vi "Save CRT data to file.vi"(5 "GPS data granularity (minutes)":refnum<vi>, 6 "Hitrate save info":T2, 7 "ROB data granularity (minutes)":refnum<vi>, 8 "error in":errorcluster, 9 "Run ID":refnum<vi>, 10 "ROB Info cluster":refnum<vi>, 11 "HDF5 data file":refnum<vi>) -> (0 "error out":errorcluster)   [LabVIEW 2016]
uses:
  Typedefs/Hit chart cluster refnum.ctl
  Typedefs/CoincidencesToSave.ctl
  Typedefs/CoincidenceWithGPSformat.ctl
  Global Variables/take CRT data.vi
  <vilib>/addons/h5labview2/group/H5G.lvlib
  <vilib>/addons/h5labview2/dataset/H5D.lvlib
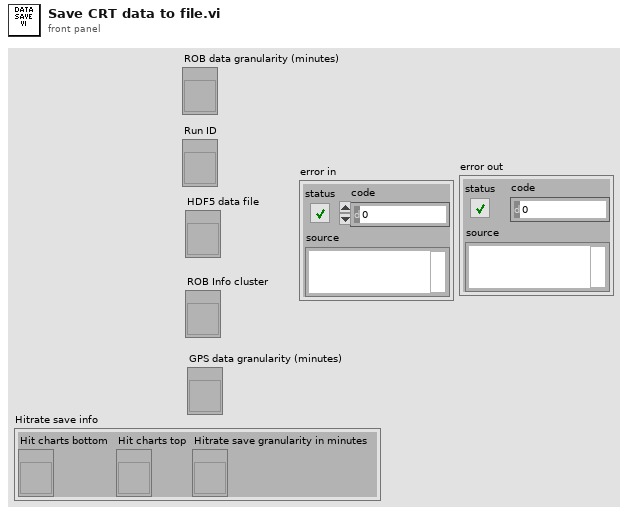
[diagram p1: front panel]
types:
  T1 = typedef "Hit chart cluster refnum.ctl" = refnum<vi>
  T2 = cluster{"Hit charts bottom":T1, "Hit charts top":T1, "Hitrate save granularity in minutes":refnum<vi>}
  T3 = typedef "CoincidenceWithGPSformat.ctl" = cluster{"Low-res hit time":u32, "Hi-res hit time":u32, "Secondary ID":i8, "DeltaT":i32, "Primary ID":i8}
  T4 = typedef "CoincidencesToSave.ctl" = T3[]
  T5 = cluster{"Timestamp":u32, "Fix quality":i8, "Satelites":i8}
  T6 = enum16{"insertPPS", "insertUTC", "read", "initiate"}
  T7 = typedef "hid_t.ctl" = i32
  T8 = cluster{"Pixel":i8, "Hi res hit time":u32, "Low res hit time":u32, "DeltaT":i16}[]
  T9 = typedef "HitChart.ctl" = cluster{"Waveform Chart":cluster{"Coincidences":dbl, "Non-coincidences":dbl, "Ratio":dbl, "Total hits":dbl}[], "Last update timestamp":timestamp, "Resolution(s)":dbl, "nondisplayed coincs":i32, "nondisplayed noncoincs":i32, "Last upd":i64, "ID":i8}
  T10 = cluster{"Waveform Chart":T9, "Waveform Chart 2":T9, "Waveform Chart 3":T9, "Waveform Chart 4":T9, "Waveform Chart 5":T9, "Waveform Chart 6":T9, "Waveform Chart 7":T9, "Waveform Chart 8":T9}
  T11 = cluster{"timestamp":u32, "ch0":dbl, "ch1":dbl, "ch2":dbl, "ch3":dbl, "ch4":dbl, "ch5":dbl, "ch6":dbl, "ch7":dbl, "ch8":dbl, "ch9":dbl, "ch10":dbl, "ch11":dbl, "ch12":dbl, "ch13":dbl, "ch14":dbl, "ch15":dbl}[]
  T12 = cluster{"Timestamp":u32, "Fix quality":i8, "Satelites":i8}[]
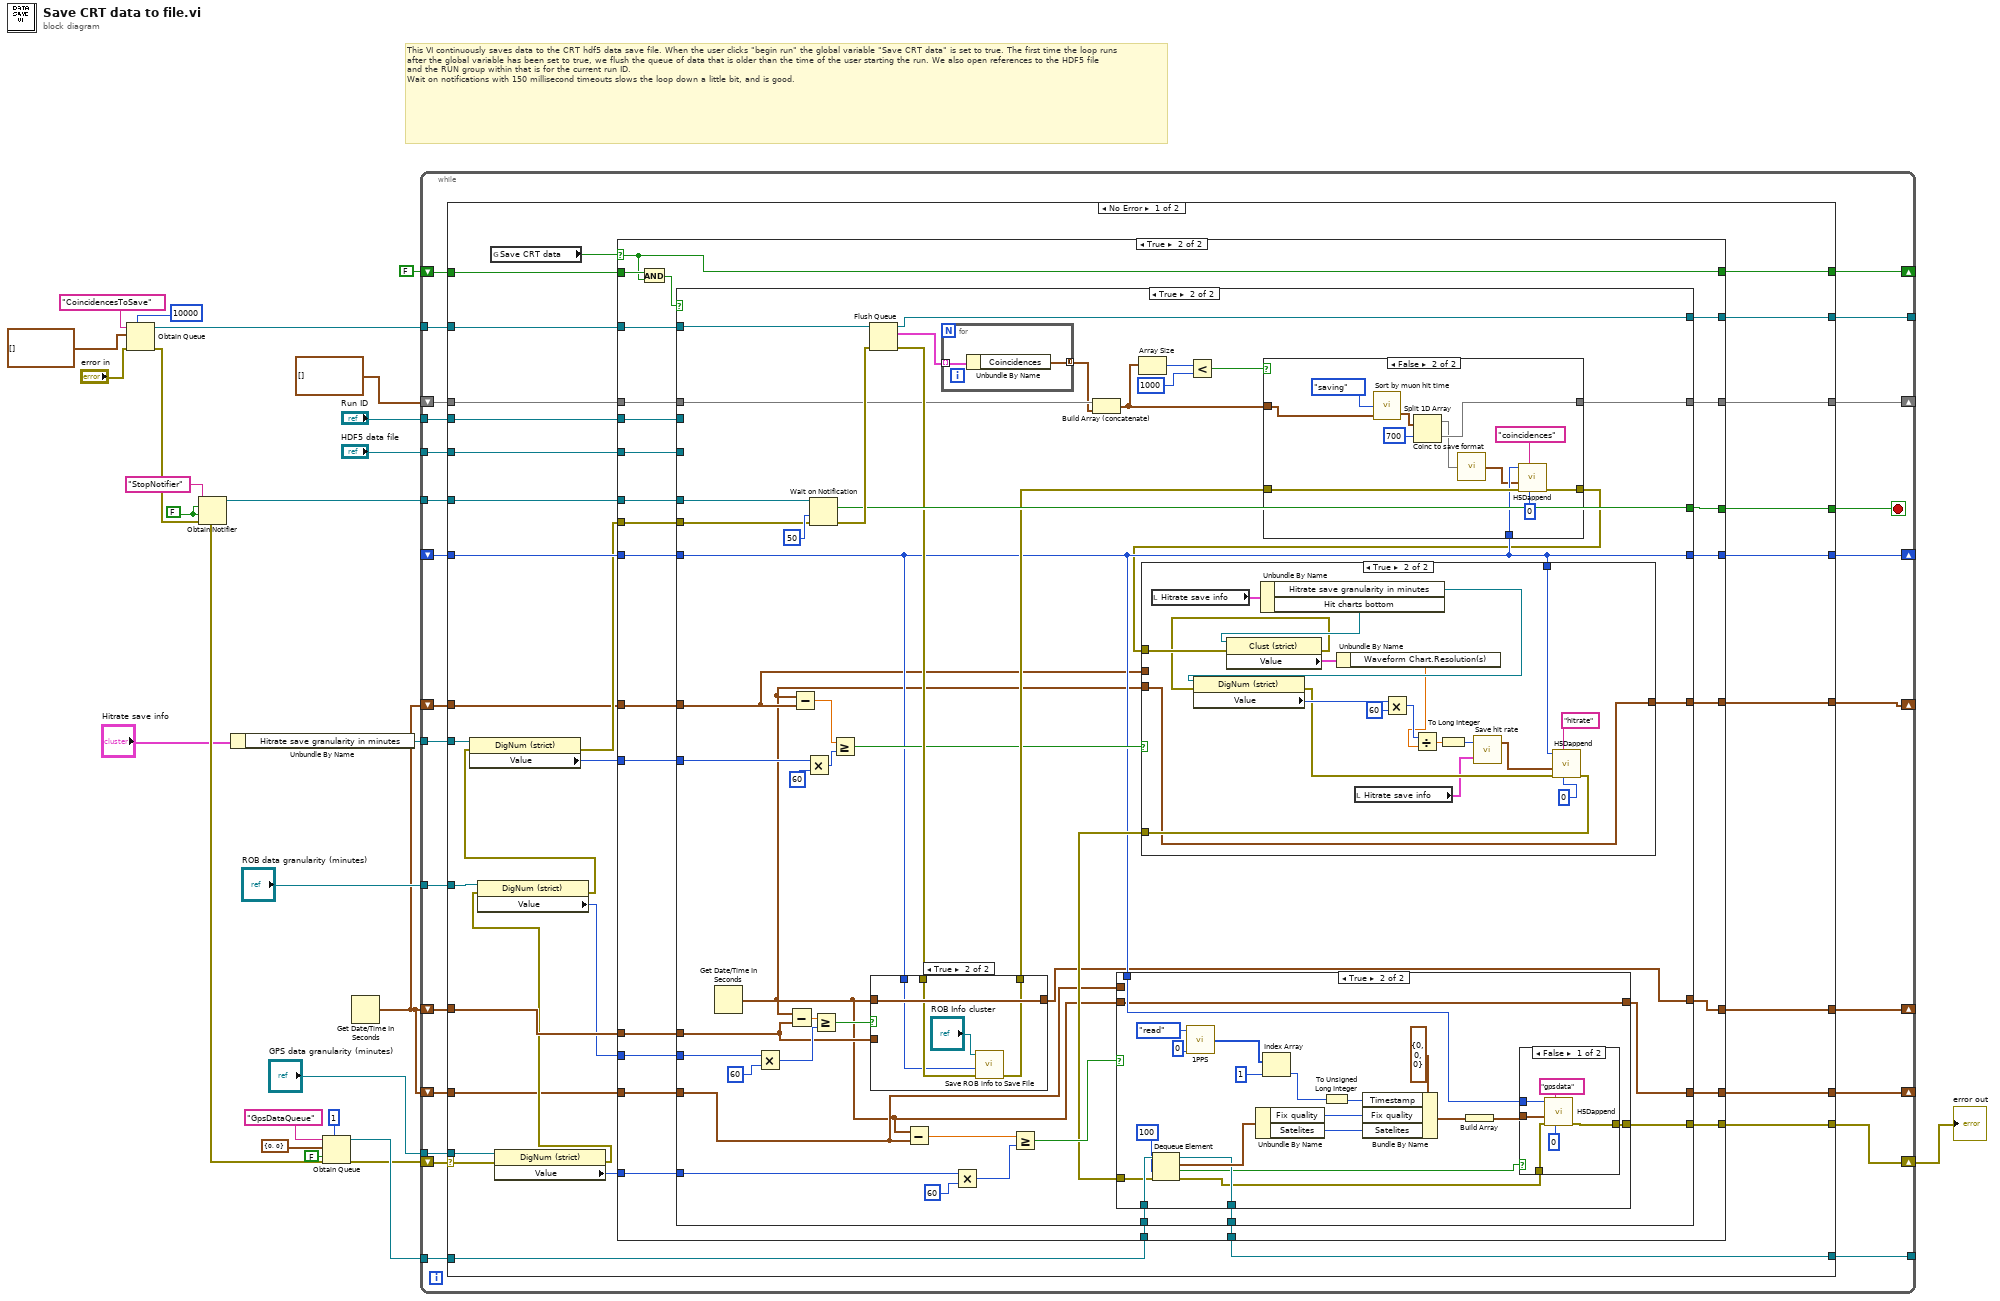
[diagram p0: block diagram]
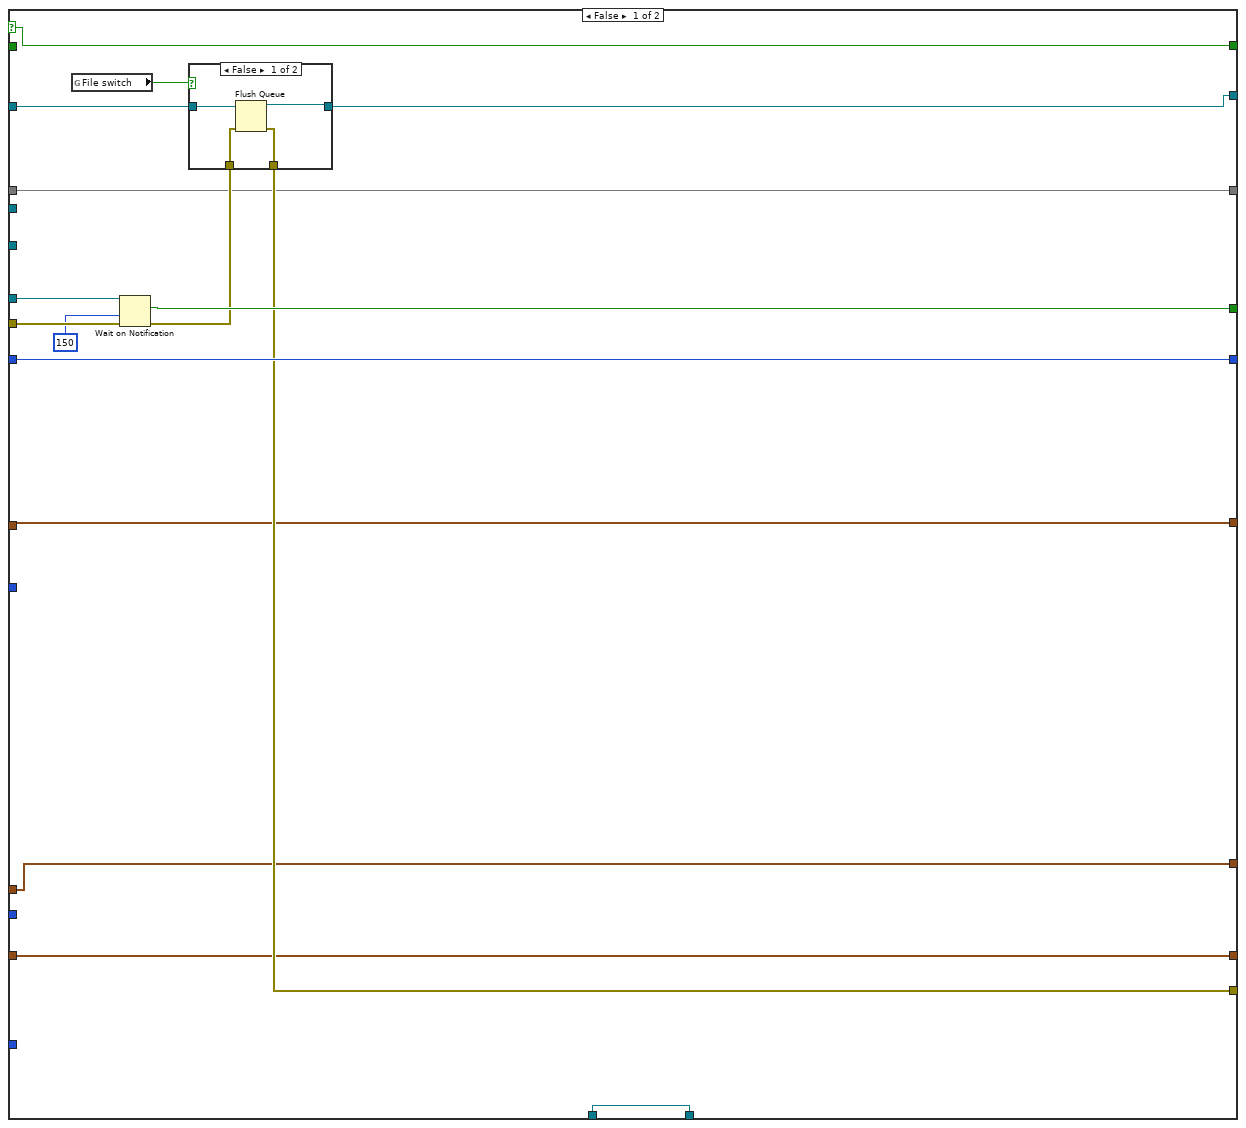
[diagram p2: hidden frame]
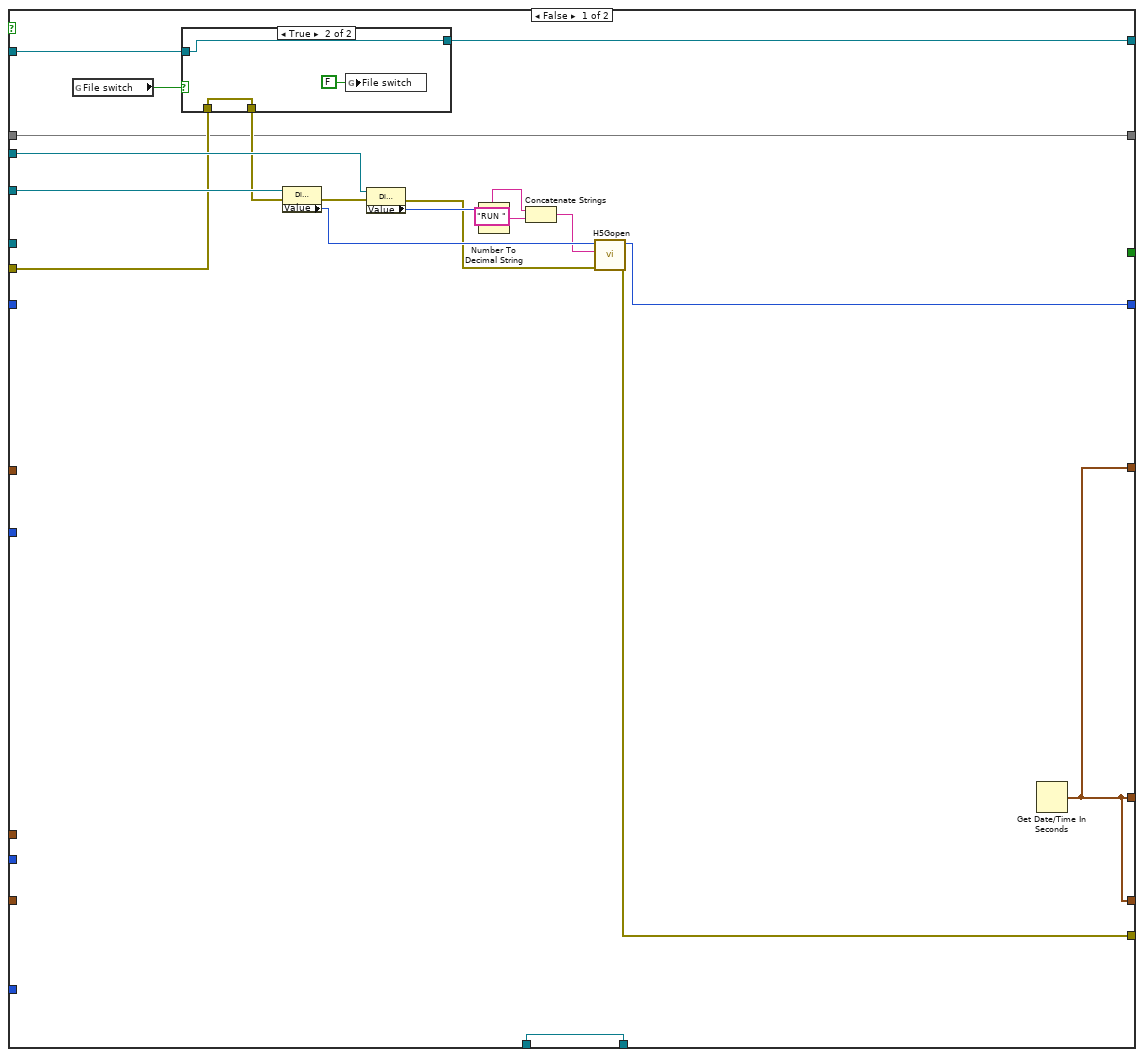
[diagram p4: hidden frame]
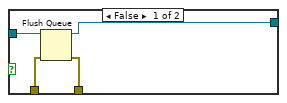
[diagram p5: hidden frame]
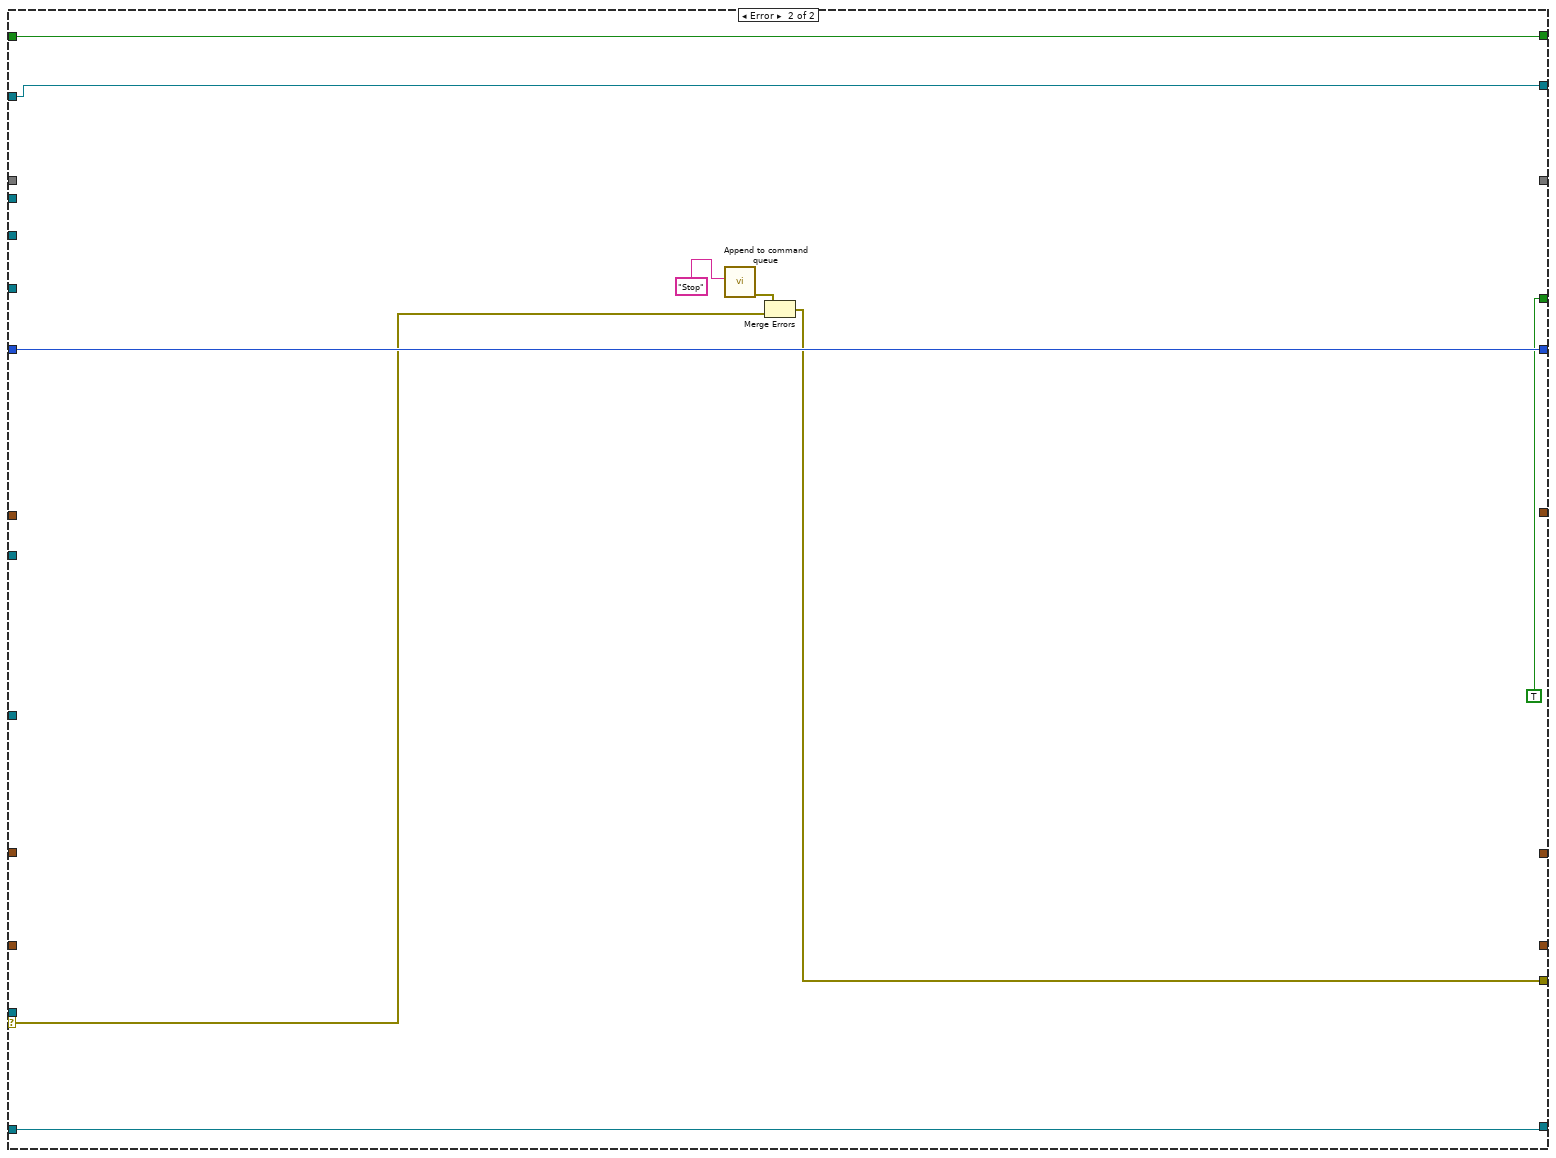
[diagram p11: hidden frame]
diagram:
  w19 = FALSE
  # "This VI continuously saves data to the CRT hdf5 data save file. When the user clicks \"begin run\" the global variable \"Save CRT data\" is set to true. The first time the loop runs after the global variable has been set to true, we flush the queue of data that is older than the time of the user starting the run. We also open references to the HDF5 file and the RUN group within that is for the current run ID.\nWait on notifications with 150 millisecond timeouts slows the loop down a little bit, and is good."
  n1 = Obtain Queue(max queue size (-1, unlimited)=10000, name (unnamed)="CoincidencesToSave", element data type=T4 [] ("Coincidences"), error in (no error)="error in") -> (queue out=w24:refnum<queue>, error out=w9:errorcluster)  [unwired: 1 in, 1 out]
  n2 = Obtain Notifier(name (unnamed)="StopNotifier", notification data type=w19, create if not found? (T)=w19, error in (no error)=w9) -> (notifier out=w18:refnum<notifier>, error out=w4:errorcluster)  [unwired: 1 out]
  n3 = Unbundle By Name("Hitrate save info") -> ("Hitrate save granularity in minutes"=w2:refnum<vi>)
  n4 = Obtain Queue(max queue size (-1, unlimited)=1, name (unnamed)="GpsDataQueue", element data type=cluster{"Fix quality":i8, "Satelites":i8} {"Fix quality"=0, "Satelites"=0}, create if not found? (T)=FALSE, error in (no error)=w4) -> (queue out=w8:refnum<queue>, error out=w6:errorcluster)  [unwired: 1 out]
  n5 = Get Date/Time In Seconds() -> (seconds since 1Jan1904=w1:timestamp)
  n6 = while {
    shift-right: [w51] -> _
    shift-left: FALSE -> [w50]
    tunnel: w24 -> [w49]
    shift-right: [w46] -> w17
    shift-left: w6 -> [w32]
    tunnel: "HDF5 data file" -> [w48]
    tunnel: "Run ID" -> [w47]
    shift-right: [w45] -> _
    shift-left: _ -> [w44]
    tunnel: w18 -> [w43]
    shift-right: [w39] -> _
    shift-left: w1 -> [w41]
    tunnel: "ROB data granularity (minutes)" -> [w40]
    shift-right: [w38] -> _
    shift-left: T3[] [] ("Coincidences") -> [w37]
    tunnel: "GPS data granularity (minutes)" -> [w36]
    tunnel: w8 -> [w35]
    tunnel: [w34] -> _
    tunnel: [w33] -> _
    tunnel: w2 -> [w31]
    shift-right: [w28] -> _
    shift-left: w1 -> [w30]
    shift-right: [w27] -> _
    shift-left: w1 -> [w29]
    stop <- w42 stop-if-true
    n7 = case shown="No Error" w32 {
      selector: w32 -> [w61 w283]
      tunnel: [w82 w286] -> w51
      tunnel: w50 -> [w81 w286]
      tunnel: w49 -> [w80 w279]
      tunnel: w48 -> [w79 _]
      tunnel: w47 -> [w78 _]
      tunnel: [w77 w282] -> w46
      tunnel: [w76 w287] -> w45
      tunnel: w44 -> [w75 w287]
      tunnel: w43 -> [w74 _]
      tunnel: [w73 TRUE] -> w42
      tunnel: w41 -> [w72 _]
      tunnel: w40 -> [w71 _]
      tunnel: [w69 _] -> w39
      tunnel: [w68 _] -> w38
      tunnel: w37 -> [w67 _]
      tunnel: w36 -> [w66 _]
      tunnel: w35 -> [w64 w280]
      tunnel: [w63 w279] -> w34
      tunnel: [w62 w280] -> w33
      tunnel: w31 -> [w59 _]
      tunnel: w30 -> [w55 _]
      tunnel: w29 -> [w54 _]
      tunnel: [w53 _] -> w28
      tunnel: [w52 _] -> w27
      frame No Error {
        n8 = global read "take CRT data.vi" "Save CRT data"() -> (w83:bool)
        n9 = property class="DigNum (strict)"(reference=w66, error in=w61) -> (error out=w60:errorcluster, "Value"=w65:i32)  [unwired: 1 out]
        n10 = property class="DigNum (strict)"(reference=w71, error in=w60) -> (error out=w58:errorcluster, "Value"=w70:i32)  [unwired: 1 out]
        n11 = property class="DigNum (strict)"(reference=w59, error in=w58) -> (error out=w56:errorcluster, "Value"=w57:i32)  [unwired: 1 out]
        n12 = case shown="True" w83 {
          selector: w83 -> [w91 w130]
          tunnel: [w91 w130] -> w82
          tunnel: w81 -> [_ w131]
          tunnel: w80 -> [w94 w128]
          tunnel: w56 -> [w98 w127]
          tunnel: w79 -> [_ w126]
          tunnel: w78 -> [_ w125]
          tunnel: [w92 w124] -> w77
          tunnel: [w99 w123] -> w76
          tunnel: w75 -> [w99 w122]
          tunnel: w74 -> [w97 w121]
          tunnel: [w95 w120] -> w73
          tunnel: w72 -> [w90 w119]
          tunnel: w70 -> [_ w118]
          tunnel: [w90 w117] -> w69
          tunnel: [w89 w116] -> w68
          tunnel: w67 -> [w89 w115]
          tunnel: w65 -> [_ w114]
          tunnel: w64 -> [w87 w113]
          tunnel: [w86 w112] -> w63
          tunnel: [w87 w111] -> w62
          tunnel: w57 -> [_ w110]
          tunnel: w55 -> [w85 w109]
          tunnel: w54 -> [w84 w108]
          tunnel: [w85 w107] -> w53
          tunnel: [w84 w106] -> w52
          frame False {
            n13 = global read "take CRT data.vi" "File switch"() -> (w88:bool)
            n14 = Wait on Notification(notifier=w97, timeout in ms (-1)=150, error in (no error)=w98) -> (notification=w95:bool, error out=w93:errorcluster)  [unwired: 1 in, 2 out]
            n15 = case shown="False" w88 {
              tunnel: w94 -> [w103 w104]
              tunnel: w93 -> [w102 w105]
              tunnel: [w101 w105] -> w92
              tunnel: [w100 w104] -> w86
              frame False {
                n16 = Flush Queue(queue=w103, error in (no error)=w102) -> (queue out=w100:refnum<queue>, error out=w101:errorcluster)  [unwired: 1 out]
              }
              frame True {
              }
            }
          }
          frame True {
            n17 = And(x=w131, y=w130) -> (x .and. y?=w129:bool)
            n18 = case shown="True" w129 {
              tunnel: w128 -> [w150 w202]
              tunnel: w127 -> [w139 w199]
              tunnel: w126 -> [w149 _]
              tunnel: w125 -> [w147 _]
              tunnel: [w137 w174] -> w124
              tunnel: [w140 w168] -> w123
              tunnel: w122 -> [_ w168]
              tunnel: w121 -> [_ w197]
              tunnel: [_ w196] -> w120
              tunnel: w119 -> [_ w179]
              tunnel: w118 -> [_ w195]
              tunnel: [w132 w163] -> w117
              tunnel: [w136 w187] -> w116
              tunnel: w115 -> [w136 w189]
              tunnel: w114 -> [_ w178]
              tunnel: w113 -> [w134 w177]
              tunnel: [w133 w176] -> w112
              tunnel: [w134 w175] -> w111
              tunnel: w110 -> [_ w172]
              tunnel: w109 -> [_ w161]
              tunnel: w108 -> [_ w159]
              tunnel: [w132 w162] -> w107
              tunnel: [w132 w160] -> w106
              frame False {
                n19 = global read "take CRT data.vi" "File switch"() -> (w135:bool)
                n20 = case shown="True" w135 {
                  tunnel: w150 -> [w154 w155]
                  tunnel: w139 -> [w153 w157]
                  tunnel: [w152 w157] -> w138
                  tunnel: [w151 w155] -> w133
                  frame False {
                    n21 = Flush Queue(queue=w154, error in (no error)=w153) -> (queue out=w151:refnum<queue>, error out=w152:errorcluster)  [unwired: 1 out]
                  }
                  frame True {
                    n22 = global write "take CRT data.vi" "File switch"(FALSE ("File switch")) -> ()
                  }
                }
                n23 = property class="DigNum (strict)"(reference=w149, error in=w138) -> (error out=w148:errorcluster, "Value"=w146:T7)  [unwired: 1 out]
                n24 = property class="DigNum (strict)"(reference=w147, error in=w148) -> (error out=w141:errorcluster, "Value"=w145:i32)  [unwired: 1 out]
                n25 = Number To Decimal String(number=w145) -> (decimal integer string=w143:string)  [unwired: 1 in]
                n26 = Concatenate Strings("RUN ", w143) -> (w142:string)
                n27 = call <vilib>:"H5Gopen.vi"("error in (no error)"=w141, "name"=w142, "ref in"=w146) -> ("error out"=w137:errorcluster, "group out"=w140:T7)  [unwired: 7 in]
                n28 = Get Date/Time In Seconds() -> (seconds since 1Jan1904=w132:timestamp)
              }
              frame True {
                n29 = Get Date/Time In Seconds() -> (seconds since 1Jan1904=w158:timestamp)
                n30 = Multiply(x=w195, y=60) -> (x*y=w193:i32)
                n31 = Subtract(x=w158, y=w179) -> (x-y=w166:dbl)
                n32 = Subtract(x=w158, y=w159) -> (x-y=w164:dbl)
                n33 = Multiply(x=w172, y=60) -> (x*y=w171:i32)
                n34 = Wait on Notification(notifier=w197, timeout in ms (-1)=50, error in (no error)=w199) -> (notification=w196:bool, error out=w198:errorcluster)  [unwired: 1 in, 2 out]
                n35 = Greater Or Equal?(x=w166, y=w193) -> (x >= y?=w190:bool)
                n36 = Greater Or Equal?(x=w164, y=w171) -> (x >= y?=w170:bool)
                n37 = Flush Queue(queue=w202, error in (no error)=w198) -> (queue out=w176:refnum<queue>, remaining elements=w201:cluster{"Coincidences":T4}[], error out=w192:errorcluster)
                n38 = case shown="True" w190 {
                  tunnel: w192 -> [w257 w259]
                  tunnel: w168 -> [_ w258]
                  tunnel: [w257 w260] -> w191
                  tunnel: w158 -> [_ w261]
                  tunnel: w179 -> [w256 _]
                  tunnel: [w256 w261] -> w163
                  frame False {
                  }
                  frame True {
                    n39 = call "Save ROB info to Save File.vi"("error in (no error)"=w259, "Fileref"=w258, "ROB info clusters"="ROB Info cluster") -> ("error out"=w260:errorcluster)  [unwired: 8 in]
                  }
                }
                n40 = Subtract(x=w158, y=w161) -> (x-y=w165:dbl)
                n41 = for {
                  tunnel: w201 -> [w278] mode=indexing
                  tunnel: [w277] -> w188 mode=concatenating
                  n42 = Unbundle By Name(w278) -> ("Coincidences"=w277:T4)
                }
                n43 = Multiply(x=w178, y=60) -> (x*y=w182:i32)
                n44 = Greater Or Equal?(x=w165, y=w182) -> (x >= y?=w180:bool)
                n45 = Build Array (concatenate)(w189, w188) -> (w186:T4)
                n46 = Array Size(array=w186) -> (size(s)=w185:i32)
                n47 = Less?(x=w185, y=1000) -> (x < y?=w183:bool)
                n48 = case shown="False" w183 {
                  tunnel: w191 -> [w264 w276]
                  tunnel: [w264 w275] -> w167
                  tunnel: w168 -> [_ w274]
                  tunnel: [w263 w269] -> w187
                  tunnel: w186 -> [w263 w266]
                  frame True {
                  }
                  frame False {
                    n49 = call "Sort by muon hit time.vi"("Top Coincs saving"=w266, "Type"=enum16{"internal", "saving"}."saving") -> ("Coincidences saving"=w270:T4)  [unwired: 1 in, 1 out]
                    n50 = Split 1D Array(array=w270, index=700) -> (first subarray=w268:T4, second subarray=w269:T4)
                    n51 = call "Coinc to save format.vi"("Coincidences"=w268) -> ("Array"=w267:T8)
                    n52 = call <vilib>:"H5Dappend.vi"("axis (first)"=0, "dataset name"="coincidences", "error in (no error)"=w276, "data"=w267, "ref in"=w274) -> ("error out"=w275:errorcluster)  [unwired: 3 in, 3 out]
                  }
                }
                n53 = case shown="True" w170 {
                  tunnel: [w204 w214] -> w169
                  tunnel: w168 -> [_ w213]
                  tunnel: w167 -> [w204 w209]
                  tunnel: [w203 w206] -> w160
                  tunnel: w159 -> [w203 _]
                  tunnel: w158 -> [_ w206]
                  frame False {
                  }
                  frame True {
                    n54 = local read "Hitrate save info"() -> (w219:T2)
                    n55 = Unbundle By Name(w219) -> ("Hitrate save granularity in minutes"=w224:refnum<vi>, "Hit charts bottom"=w212:T1)
                    n56 = property class="Clust (strict)"(reference=w212, error in=w209) -> (error out=w208:errorcluster, "Value"=w211:T10)  [unwired: 1 out]
                    n57 = property class="DigNum (strict)"(reference=w224, error in=w208) -> (error out=w207:errorcluster, "Value"=w223:i32)  [unwired: 1 out]
                    n58 = Unbundle By Name(w211) -> ("Waveform Chart.Resolution(s)"=w210:dbl)
                    n59 = local read "Hitrate save info"() -> (w205:T2)
                    n60 = Multiply(x=w223, y=60) -> (x*y=w221:i32)
                    n61 = Divide(x=w221, y=w210) -> (x/y=w220:dbl)
                    n62 = To Long Integer(number=w220) -> (32bit integer=w218:i32)
                    n63 = call "Save hit rate.vi"("Data cluster"=w205, "Elements to average"=w218) -> ("data"=w215:T11)  [unwired: 1 in]
                    n64 = call <vilib>:"H5Dappend.vi"("axis (first)"=0, "dataset name"="hitrate", "error in (no error)"=w207, "data"=w215, "ref in"=w213) -> ("error out"=w214:errorcluster)  [unwired: 3 in, 3 out]
                  }
                }
                n65 = case shown="True" w180 {
                  tunnel: [w225 w228] -> w162
                  tunnel: w158 -> [_ w228]
                  tunnel: w168 -> [_ w235]
                  tunnel: w169 -> [w227 w243]
                  tunnel: [w227 w240] -> w174
                  tunnel: w177 -> [w226 w244]
                  tunnel: [w226 w241] -> w175
                  tunnel: w161 -> [w225 _]
                  frame False {
                  }
                  frame True {
                    n66 = Dequeue Element(queue=w244, timeout in ms (-1)=100, error in (no error)=w243) -> (queue out=w241:refnum<queue>, element=w242:cluster{"Fix quality":i8, "Satelites":i8}, timed out?=w233:bool, error out=w236:errorcluster)
                    n67 = call "1PPS.vi"("Read Index\nNumber"=0 ("Read Index\nNumber"), "Action"=T6."read") -> ("Array"=w248:u32[])  [unwired: 2 in]
                    n68 = Unbundle By Name(w242) -> ("Fix quality"=w239:i8, "Satelites"=w238:i8)
                    n69 = Index Array(array=w248, index=1) -> (element=w230:u32)
                    n70 = To Unsigned Long Integer(number=w230) -> (unsigned 32bit integer=w229:u32)
                    n71 = Bundle By Name(cluster=T5 {"Timestamp"=0, "Fix quality"=0, "Satelites"=0} ("output cluster"), "Timestamp"=w229, "Fix quality"=w239, "Satelites"=w238) -> (w232:T5)
                    n72 = Build Array(w232) -> (w231:T12)
                    n73 = case shown="False" w233 {
                      tunnel: [w253 w255] -> w240
                      tunnel: w231 -> [w252 _]
                      tunnel: w236 -> [w251 w255]
                      tunnel: w235 -> [w250 _]
                      frame False {
                        n74 = call <vilib>:"H5Dappend.vi"("axis (first)"=0, "dataset name"="gpsdata", "error in (no error)"=w251, "data"=w252, "ref in"=w250) -> ("error out"=w253:errorcluster)  [unwired: 3 in, 3 out]
                      }
                      frame True {
                      }
                    }
                  }
                }
              }
            }
          }
        }
      }
      frame Error {
        n75 = call "Append to command queue.vi"("Single command"="Stop") -> ("error out"=w284:errorcluster)  [unwired: 10 in]
        n76 = Merge Errors(w284, w283) -> (w282:errorcluster)
      }
    }
  }
  "error out" <- w17
